vi "2-Degree centrigade to Fahrenheit.vi"() -> ()   [LabVIEW 2019]
panel:
  out "Temperature in Celsius":dbl(slide)=37.0 scale=0.0..200.0
  out "Temperature in Fahrenheit":dbl(slide)=98.60000000000001 scale=0.0..200.0
  in  "?":bool
  out "?":dbl=98.60000000000001
  in  "?":dbl=37.0
  # "DEGREE CENTIGRADE TO FAHRENHEIT"
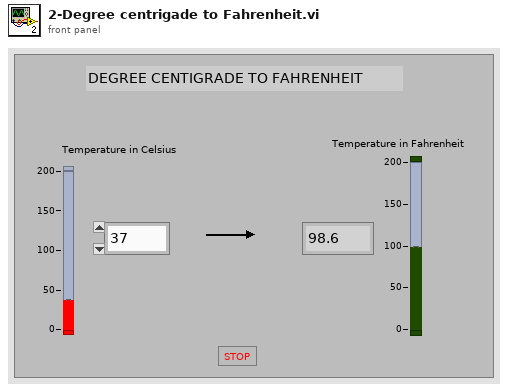
[diagram p1: front panel]
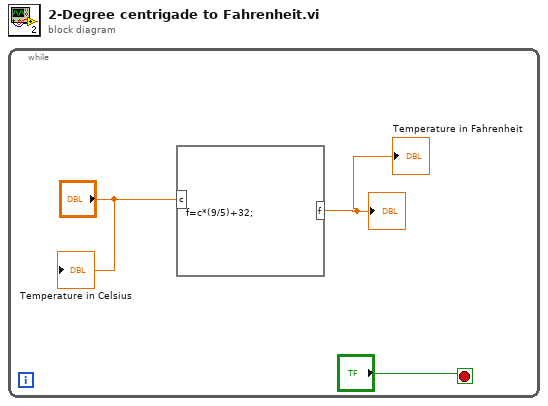
[diagram p0: block diagram]
diagram:
  n1 = while {
    stop <- "?" stop-if-true
    n2 = formula code="f=c*(9/5)+32;"("c"="?") -> ("f"=→"?" →"Temperature in Fahrenheit":dbl)
    "Temperature in Celsius" <- "?"
  }
